vi "CamGetMinMaxExpo.vi"(8 "error in (no error)":errorcluster, 11 "hCam":i16) -> (0 "error in (no error) 2":errorcluster, 2 "output cluster":cluster{"Range.min":u32, "Range.max":u32}, 3 "hCam out":i16)   [LabVIEW 2021]
panel:
  in  "Cluster":cluster{"Range.min":u32, "Range.max":u32}
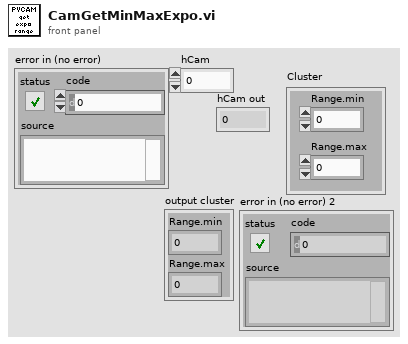
[diagram p1: front panel]
types:
  T1 = enum16{"ATTR_CURRENT", "ATTR_COUNT", "ATTR_TYPE", "ATTR_MIN", "ATTR_MAX", "ATTR_DEFAULT", "ATTR_INCREMENT", "ATTR_ACCESS", "ATTR_AVAIL"}
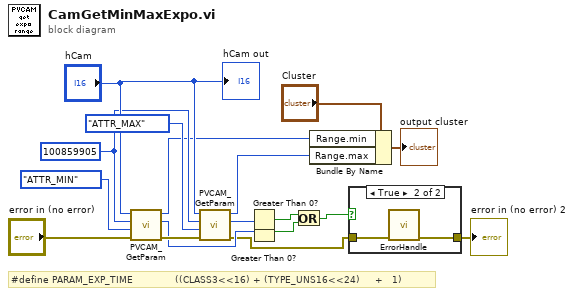
[diagram p0: block diagram]
diagram:
  w13 = u32 100859905 ("param_id")
  # "#define PARAM_EXP_TIME              ((CLASS3<<16) + (TYPE_UNS16<<24)     +   1)"
  n1 = call "PVCAM_GetParam.vi"("error in (no error)"="error in (no error)", "param_attrib"=T1."ATTR_MIN", "param_id"=w13, "hCam"="hCam") -> ("error out"=w15:errorcluster, "return type"=w7:i16, "param_value"=w10:u16)  [unwired: 5 in]
  n2 = call "PVCAM_GetParam.vi"("error in (no error)"=w15, "param_attrib"=T1."ATTR_MAX", "param_id"=w13, "hCam"="hCam") -> ("error out"=w3:errorcluster, "return type"=w8:i16, "param_value"=w9:u16)  [unwired: 5 in]
  n3 = Greater Than 0?(x=w8) -> (x > 0?=w5:bool)
  n4 = Greater Than 0?(x=w7) -> (x > 0?=w6:bool)
  n5 = Or(x=w5, y=w6) -> (x .or. y?=w4:bool)
  n6 = Bundle By Name(cluster="Cluster", "Range.min"=w10, "Range.max"=w9) -> (→"output cluster":cluster{"Range.min":u32, "Range.max":u32})
  n7 = case shown="True" w4 {
    tunnel: w3 -> [w18 w20]
    tunnel: [w18 w19] -> w2
    frame False {
    }
    frame True {
      n8 = call "ErrorHandle.vi"("error in (no error)"=w20) -> ("error in (no error) 2"=w19:errorcluster)  [unwired: 10 in]
    }
  }
  "error in (no error) 2" <- w2
  "hCam out" <- "hCam"
